vi "Do.vi"(8 "error in (no error)":errorcluster, 10 "Actor in":refnum<class "Actor.lvclass">, 11 "Read Multi-Point [MP] Msg":refnum<class "Read Multi-Point [MP] Msg.lvclass">) -> (0 "error out":errorcluster, 2 "Actor out":refnum<class "Actor.lvclass">)   [LabVIEW 2016, in "CS++DMM.lvlib" / "Read Multi-Point [MP] Msg.lvclass"]
doc: "This VI delivers the message to the actor by calling the appropriate method(s) on the actor."
uses:
  Read Multi-Point [MP] Msg.lvclass
  <vilib>/ActorFramework/Actor/Actor.lvclass
  C:/User/Brand/LVP/CSPP-Dev/Packages/CSPP_Core/Actors/CS++PVMonitor Messages/CS++PVUpdate Msg/CS++PVUpdate Msg.lvclass
  CS++DMM/CS++DMM.lvclass
  C:/Program Files (x86)/National Instruments/LabVIEW 2016/vi.lib/ActorFramework/Actor/Actor.lvclass
  CSPP_Core/Actors/CS++PVMonitor Messages/CS++PVUpdate Msg/CS++PVUpdate Msg.lvclass/CS++PVUpdate Msg.ctl
  CSPP_Core/Classes/CS++ProcessVariables/ProcessVariable/PV.lvclass/PV.ctl
  Read Multi-Point [MP] Msg.lvclass/Read Multi-Point [MP] Msg.ctl
  CSPP_Core/Classes/CS++ProcessVariables/ProcessVariable/PV.lvclass
  CSPP_Core/Actors/CS++PVMonitor Messages/CS++PVUpdate Msg/CS++PVUpdate Msg.lvclass
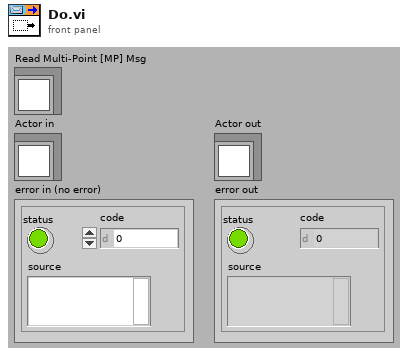
[diagram p1: front panel]
types:
  T1 = cluster{"maximum time (5s)":dbl[unit], "array size":i32}
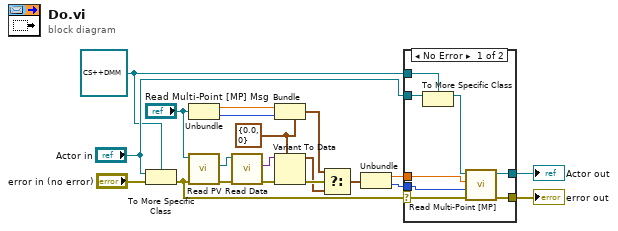
[diagram p0: block diagram]
diagram:
  w12 = T1 {"maximum time (5s)"=0.0, "array size"=0} ("Type")
  w16 = refnum<class "CS++DMM.lvclass"> refnum ("Actor in")
  n1 = To More Specific Class(target class=w16, reference="Actor in", error in="error in (no error)") -> (error out=w5:errorcluster)  [unwired: 1 out]
  n2 = Unbundle ("Pre-Unbundler")("Read Multi-Point [MP] Msg") -> (w3:dbl[unit], w2:i32)
  n3 = call "Read PV.vi"("error in (no error)"=w5, "CS++PVUpdate Msg in"="Read Multi-Point [MP] Msg") -> ("error out"=w15:errorcluster, "PV"=w11:refnum<class "PV.lvclass">)  [unwired: 7 in, 1 out]
  n4 = call "Read Data.vi"("error in (no error)"=w15, "PV in"=w11) -> ("error out"=w9:errorcluster, "Data"=w10:variant)  [unwired: 7 in, 1 out]
  n5 = Bundle ("Pre-Bundler")(cluster=w12, "maximum time (5s)"=w3, "array size"=w2) -> (w13:T1)
  n6 = Variant To Data(error in=w9, type=w12, Variant=w10) -> (data=w7:T1, error out=w14:errorcluster)
  n7 = Select ("MainSelect")(t=w13, s=w14, f=w7) -> (s? t:f=w8:T1)
  n8 = Unbundle ("Main-Unbundler")(w8) -> ("maximum time (5s)"=w4:dbl[unit], "array size"=w1:i32)
  n9 = case shown="No Error" w5 {
    selector: w5 -> [w26 w30]
    tunnel: [w28 w30] -> w19
    tunnel: [w27 w29] -> w18
    tunnel: "Actor in" -> [w25 w29]
    tunnel: w16 -> [w24 _]
    tunnel: w4 -> [w22 _]
    tunnel: w1 -> [w21 _]
    frame No Error {
      n10 = To More Specific Class(target class=w24, reference=w25) -> (specific class reference=w23:refnum<class "CS++DMM.lvclass">)  [unwired: 1 in, 1 out]
      n11 = call "Read Multi-Point [MP].vi"("error in (no error)"=w26, "array size"=w21, "maximum time (5s)"=w22, "CS++DMM in"=w23) -> ("error out"=w28:errorcluster, "CS++DMM out"=w27:refnum<class "CS++DMM.lvclass">)  [unwired: 4 in, 2 out]
    }
    frame Error {
    }
  }
  "error out" <- w19
  "Actor out" <- w18
